vi "[RT]NTC_calc.vi"(10 "milliseconds to wait":u32, 11 "dbl Scaled Value":dbl) -> (3 "Temp_NTC":dbl)   [LabVIEW 2018]
uses:
  [GlobVar]SensorState.vi
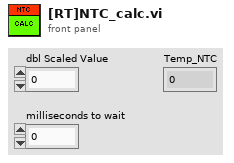
[diagram p1: front panel]
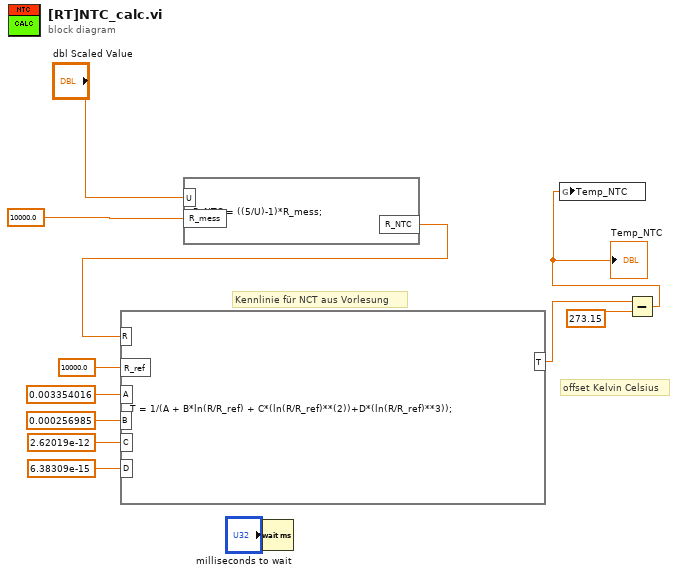
[diagram p0: block diagram]
diagram:
  # "offset Kelvin Celsius"
  # "Kennlinie für NCT aus Vorlesung"
  n1 = formula code="R_NTC = ((5/U)-1)*R_mess;"("U"="dbl Scaled Value", "R_mess"=10000.0 ("input variable")) -> ("R_NTC"=w2:dbl)
  n2 = formula code="T = 1/(A + B*ln(R/R_ref) + C*(ln(R/R_ref)**(2))+D*(ln(R/R_ref)**3));"("R_ref"=10000.0 ("input variable"), "R"=w2, "A"=0.003354016 ("input variable"), "B"=0.000256985 ("input variable"), "C"=2.62019e-12 ("input variable"), "D"=6.38309e-15 ("input variable")) -> ("T"=w11:dbl)
  n3 = Wait (ms)(milliseconds to wait="milliseconds to wait") -> ()  [unwired: 1 out]
  n4 = Subtract(x=w11, y=273.15) -> (x-y=w12:dbl)
  "Temp_NTC" <- w12
  n5 = global write "[GlobVar]SensorState.vi" "Temp_NTC"(w12) -> ()
